vi "Update Fault Indicator.vi"(8 "error in (no error)":errorcluster, 11 "DLS Laser Actor in":refnum<class "FLS Laser Actor.lvclass">) -> (0 "error out":errorcluster, 3 "DLS Laser Actor out":refnum<class "FLS Laser Actor.lvclass">)   [LabVIEW 2018, in "FLS Laser Actor.lvlib" / "FLS Laser Actor.lvclass"]
uses:
  FLS Laser Actor.lvclass
  FLS Laser Actor.lvclass/FLS Laser Actor.ctl
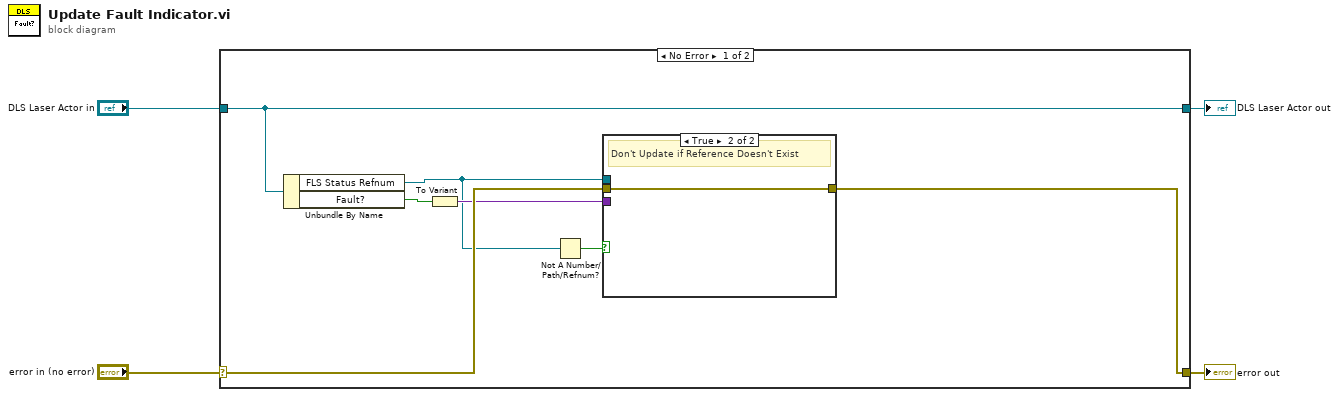
[diagram p0: block diagram]
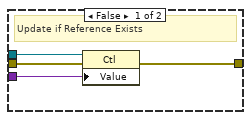
[diagram p2: hidden frame]
diagram:
  n1 = case shown="No Error" "error in (no error)" {
    selector: "error in (no error)" -> [w10 w18]
    tunnel: [w9 w18] -> w3
    tunnel: [w11 w17] -> w1
    tunnel: "DLS Laser Actor in" -> [w11 w17]
    frame No Error {
      n2 = Unbundle By Name(w11) -> ("FLS Status Refnum"=w6:refnum<vi>, "Fault?"=w8:bool)
      n3 = To Variant(anything=w8) -> (Variant=w7:variant)
      n4 = Not A Number/Path/Refnum?(number/path/refnum=w6) -> (NaN/Path/Refnum?=w5:bool)
      n5 = case shown="True" w5 {
        tunnel: w10 -> [w15 w16]
        tunnel: [w14 w16] -> w9
        tunnel: w7 -> [w13 _]
        tunnel: w6 -> [w12 _]
        frame False {
          # "Update if Reference Exists"
          n6 = property class="Ctl"(reference=w12, error in=w15, "Value"=w13) -> (error out=w14:errorcluster)  [unwired: 1 out]
        }
        frame True {
          # "Don't Update if Reference Doesn't Exist"
        }
      }
    }
    frame Error {
    }
  }
  "error out" <- w3
  "DLS Laser Actor out" <- w1
